vi "Begin.vi"(8 "error in":errorcluster) -> (0 "error out":errorcluster)   [LabVIEW 2017]
doc: "Called before other user functions, this VI is expected to open initial I/O refnums, load in file data, and do all program initialization. Notice that the <B>error out</B> terminal is simply used for data flow. Wiring it to other structures or subVIs ensures that this VI runs first."
uses:
  <vilib>/Rock Robotics/WPI/DriverStation/WPI_DriverStationRobotMode2.ctl
  <vilib>/Rock Robotics/WPI/Joystick/WPI_JoystickDeviceEnum.ctl
  <vilib>/Rock Robotics/WPI/Solenoid/WPI_SolenoidChannel.ctl
  <vilib>/Rock Robotics/SystemInterfaces/DIO/FPGA_DIORelayChannel.ctl
  <vilib>/Rock Robotics/WPI/Solenoid/WPI_SolenoidValue.ctl
  <vilib>/Rock Robotics/WPI/ThirdParty/Phoenix-LabVIEW/Motor Controller/Controls/CTRE_Phoenix_MotorControl_FeedbackDevice.ctl
  <vilib>/Rock Robotics/WPI/ThirdParty/Phoenix-LabVIEW/Motor Controller/Controls/CTRE_Phoenix_MotorControl_NeutralMode.ctl
  <vilib>/Rock Robotics/SystemInterfaces/AI/FPGA_AIChannel.ctl
  <vilib>/Rock Robotics/SystemInterfaces/DIO/FPGA_DIOChannel.ctl
  Robot Global Data.vi
  <vilib>/Rock Robotics/Network Tables/NT Write String Array.vi
  <vilib>/Rock Robotics/WPI/ThirdParty/Phoenix-LabVIEW/Pigeon IMU/CTRE_PigeonIMU_Open_TalonSRX.vi
  <vilib>/Rock Robotics/WPI/RobotDrive/WPI_RobotDriveOpen2MotorWithExistingMotors.vi
  <vilib>/Rock Robotics/WPI/Counter/WPI_CounterDigitalInputToDigitalSource.vi
  <vilib>/Rock Robotics/WPI/Solenoid/WPI_SolenoidOpenSingle.vi
  <vilib>/Rock Robotics/WPI/Solenoid/WPI_SolenoidOpenDouble.vi
  <vilib>/Rock Robotics/WPI/Utilities/WPI_GetSetVariantRefNum.vi
  <vilib>/Rock Robotics/WPI/Switch/WPI_SwitchOpenLimit.vi
  <vilib>/Rock Robotics/WPI/Solenoid/WPI_SolenoidSetEnum.vi
  <vilib>/Rock Robotics/WPI/ThirdParty/Phoenix-LabVIEW/Pigeon IMU/CTRE_PigeonIMU_Open_CAN.vi
  <vilib>/Rock Robotics/WPI/Ultrasonic/WPI_SonarMB1010DigRefNum Registry Set.vi
  <vilib>/Rock Robotics/SystemInterfaces/spilib/spi_bus.ctl
  <vilib>/Rock Robotics/WPI/Gyro/WPI_GyroXRS450_SPI_Open.vi
  <vilib>/Rock Robotics/WPI/Ultrasonic/WPI_SonarMB1010DigitalOpen.vi
panel:
  out "error out 3":errorcluster
  in  "error in 3":errorcluster
  out "error out 2":errorcluster
  in  "error in 2":errorcluster
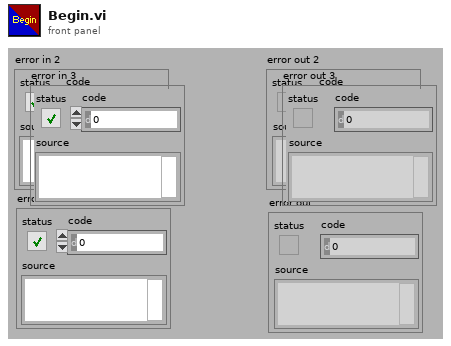
[diagram p1: front panel]
types:
  T1 = typedef "FPGA_DIOChannel.ctl" = enum8{"DIO 0", "DIO 1", "DIO 2", "DIO 3", "DIO 4", "DIO 5", "DIO 6", "DIO 7", "DIO 8", "DIO 9", "DIO MXP 0", "DIO MXP 1", "DIO MXP 2", "DIO MXP 3", "DIO MXP 4", "DIO MXP 5", "DIO MXP 6", "DIO MXP 7", "DIO MXP 8", "DIO MXP 9", "DIO MXP 10", "DIO MXP 11", "DIO MXP 12", "DIO MXP 13", "DIO MXP 14", "DIO MXP 15", "SPI Port CS1", "SPI Port CS2", "SPI Port CS3", "SPI Port MISO", "SPI Port MOSI", "Invalid"}
  T2 = typedef "WPI_JoystickDeviceEnum.ctl" = enum16{"USB 0", "USB 1", "USB 2", "USB 3", "USB 4", "USB 5"}
  T3 = typedef "WPI_SolenoidChannel.ctl" = enum8{"Solenoid 0", "Solenoid 1", "Solenoid 2", "Solenoid 3", "Solenoid 4", "Solenoid 5", "Solenoid 6", "Solenoid 7", "Invalid"}
  T4 = typedef "WPI_DriverStationRobotMode2.ctl" = enum16{"Autonomous Disabled", "Autonomous Enabled", "Teleop Disabled", "Teleop Enabled", "Disconnected", "Finish", "Test Disabled", "Test Enabled", "Emergency Stopped"}
  T5 = typedef "FPGA_AIChannel.ctl" = enum8{"AI 0", "AI 1", "AI 2", "AI 3", "AI MXP 0", "AI MXP 1", "AI MXP 2", "AI MXP 3", "Invalid"}
  T6 = typedef "CTRE_Phoenix_MotorControl_NeutralMode.ctl" = enum8{"EEPROMSetting", "Override to Coast", "Override to Brake"}
  T7 = typedef "WPI_SolenoidValue.ctl" = enum16{"Off", "On", "Forward", "Reverse"}
  T8 = typedef "FPGA_DIORelayChannel.ctl" = enum8{"Relay 0", "Relay 1", "Relay 2", "Relay 3", "Invalid"}
  T9 = typedef "spi_bus.ctl" = enum16{"SPI On-Board, CS0", "SPI On-Board, CS1", "SPI On-Board, CS2", "SPI On-Board, CS3", "SPI MXP", "Invalid"}
  T10 = typedef "WPI_JoystickDevRef.ctl" = cluster{"Device":T2}
  T11 = typedef "WPI_DigitalInputDevRef.ctl" = cluster{"DevStatus":errorcluster, "DIO Channel":T1}
  T12 = typedef "FPGA_CounterEncoderSourceConvertionLVSourceType.ctl" = cluster{"DevStatus":errorcluster, "AnalogTriggerMode?":bool, "DigitalMode":cluster{"DIO Channel":T13}, "AnalogTriggerMode":cluster{"AnalogTriggerIndex":T14, "OutputType":T15}}
  T13 = typedef "FPGA_DIODigitalSourceChannel.ctl" = enum8{"DIO 0", "DIO 1", "DIO 2", "DIO 3", "DIO 4", "DIO 5", "DIO 6", "DIO 7", "DIO 8", "DIO 9", "DIO MXP 0", "DIO MXP 1", "DIO MXP 2", "DIO MXP 3", "DIO MXP 4", "DIO MXP 5", "DIO MXP 6", "DIO MXP 7", "DIO MXP 8", "DIO MXP 9", "DIO MXP 10", "DIO MXP 11", "DIO MXP 12", "DIO MXP 13", "DIO MXP 14", "DIO MXP 15", "Disabled"}
  T14 = typedef "FPGA_AnalogTriggerIndex.ctl" = enum8{"Trig 0", "Trig 1", "Trig 2", "Trig 3", "Trig 4", "Trig 5", "Trig 6", "Trig 7", "Invalid"}
  T15 = typedef "FPGA_AnalogTriggerOutType.ctl" = enum16{"InWindow", "TriggerState", "Rising", "Falling"}
  T16 = typedef "WPI_EncoderDevRef.ctl" = cluster{"DevStatus":errorcluster, "EncoderIndex":T17, "CounterIndex":T18, "DistancePerCount":dbl, "Decoding Type":T19}
  T17 = typedef "FPGA_EncoderIdx.ctl" = enum8{"Enc 0", "Enc 1", "Enc 2", "Enc 3", "Enc 4", "Enc 5", "Enc 6", "Enc 7", "Invalid"}
  T18 = typedef "FPGA_CounterCtrSystemIndex.ctl" = enum8{"Ctr 0", "Ctr 1", "Ctr 2", "Ctr 3", "Ctr 4", "Ctr 5", "Ctr 6", "Ctr 7", "Invalid"}
  T19 = typedef "WPI_EncoderType.ctl" = enum16{"1x", "2x", "4x"}
  T20 = typedef "WPI_SolenoidDevRef.ctl" = cluster{"DevStatus":errorcluster, "Pneumatics Control Module":u8, "Forward Solenoid Channel":T3, "Reverse Solenoid Channel":T3}
  T21 = typedef "WPI_CompressorDevRef.ctl" = cluster{"DevStatus":errorcluster, "Pneumatics Control Module":u8}
  T22 = typedef "WPI_SwitchDevRef.ctl" = cluster{"DevStatus":errorcluster, "DIO Channel":T1, "CntIndex":T18, "Normally Closed":bool}
  T23 = typedef "WPI_MotorControlDeviceRef.ctl" = cluster{"DeviceStatus":errorcluster, "Type":T24, "PWM":cluster{"PWM Channel":T25, "DeadBand":T26}, "CAN":cluster{"Device Number":u8, "SetOutput VI Ref":variant, "GetOutput VI Ref":variant, "Enable VI Ref":variant, "Disable VI Ref":variant, "Data":variant}, "Invert":bool, "DIO PWM":cluster{"PWM \"Enable\" Channel":T25, "DIOChannel":T1, "PWM Rate":dbl}}
  T24 = typedef "WPI_MotorControlType.ctl" = enum16{"PWM", "CAN", "DIO PWM"}
  T25 = typedef "FPGA_DIOPWMChannel.ctl" = enum8{"PWM 0", "PWM 1", "PWM 2", "PWM 3", "PWM 4", "PWM 5", "PWM 6", "PWM 7", "PWM 8", "PWM 9", "PWM MXP 0", "PWM MXP 1", "PWM MXP 2", "PWM MXP 3", "PWM MXP 4", "PWM MXP 5", "PWM MXP 6", "PWM MXP 7", "PWM MXP 8", "PWM MXP 9", "Invalid"}
  T26 = typedef "WPI_PWMDeadband.ctl" = cluster{"Name":string, "maxPositivePwm":i32, "minPositivePwm":i32, "centerPwm":i32, "maxNegativePwm":i32, "minNegativePwm":i32, "angularRange":u16}
  T27 = typedef "WPI_RobotDriveDevRef.ctl" = cluster{"DevStatus":errorcluster, "Motors[]":T23[], "Square Inputs":bool, "Max Output":dbl}
  T28 = typedef "CTRE_PigeonIMU_DeviceRef.ctl" = cluster{"DeviceStatus":errorcluster, "Device Number":u8, "Type":T29, "Device ID":u32, "Handle":u64, "UsageFrame":u32, "Library Path":path}
  T29 = typedef "CTRE_PigeonIMU_ConnectionType.ctl" = u32
  T30 = typedef "CTRE_Phoenix_MotorControl_FeedbackDevice.ctl" = i8
  T31 = typedef "WPI_AnalogChannelDevRef.ctl" = cluster{"DevStatus":errorcluster, "Analog Channel":T5}
  T32 = typedef "WPI_SonarMB1010DigitalDeviceRef.ctl" = cluster{"CounterDevRef":T33, "Scaling factor (s/in)":dbl}
  T33 = typedef "WPI_CounterDevRef.ctl" = cluster{"DevStatus":errorcluster, "CntIndex":T18}
  T34 = typedef "WPI_RelayDevRef.ctl" = cluster{"DevStatus":errorcluster, "Relay Channel":T8, "Relay Direction":T35}
  T35 = typedef "WPI_RelayDirection.ctl" = enum16{"Both directions", "Forward only", "Reverse only"}
  T36 = typedef "WPI_GyroDevRef.ctl" = cluster{"DevStatus":errorcluster, "Analog Channel":T5, "Gain (VoltsPerDegree/Second)":dbl, "Gyro Type":enum16{"Analog", "XRS450"}, "Handle":i32, "SPI Bus":T9, "Device Found":bool, "Sample Rate":dbl, "Calibrate On Open":bool, "Offset":dbl}
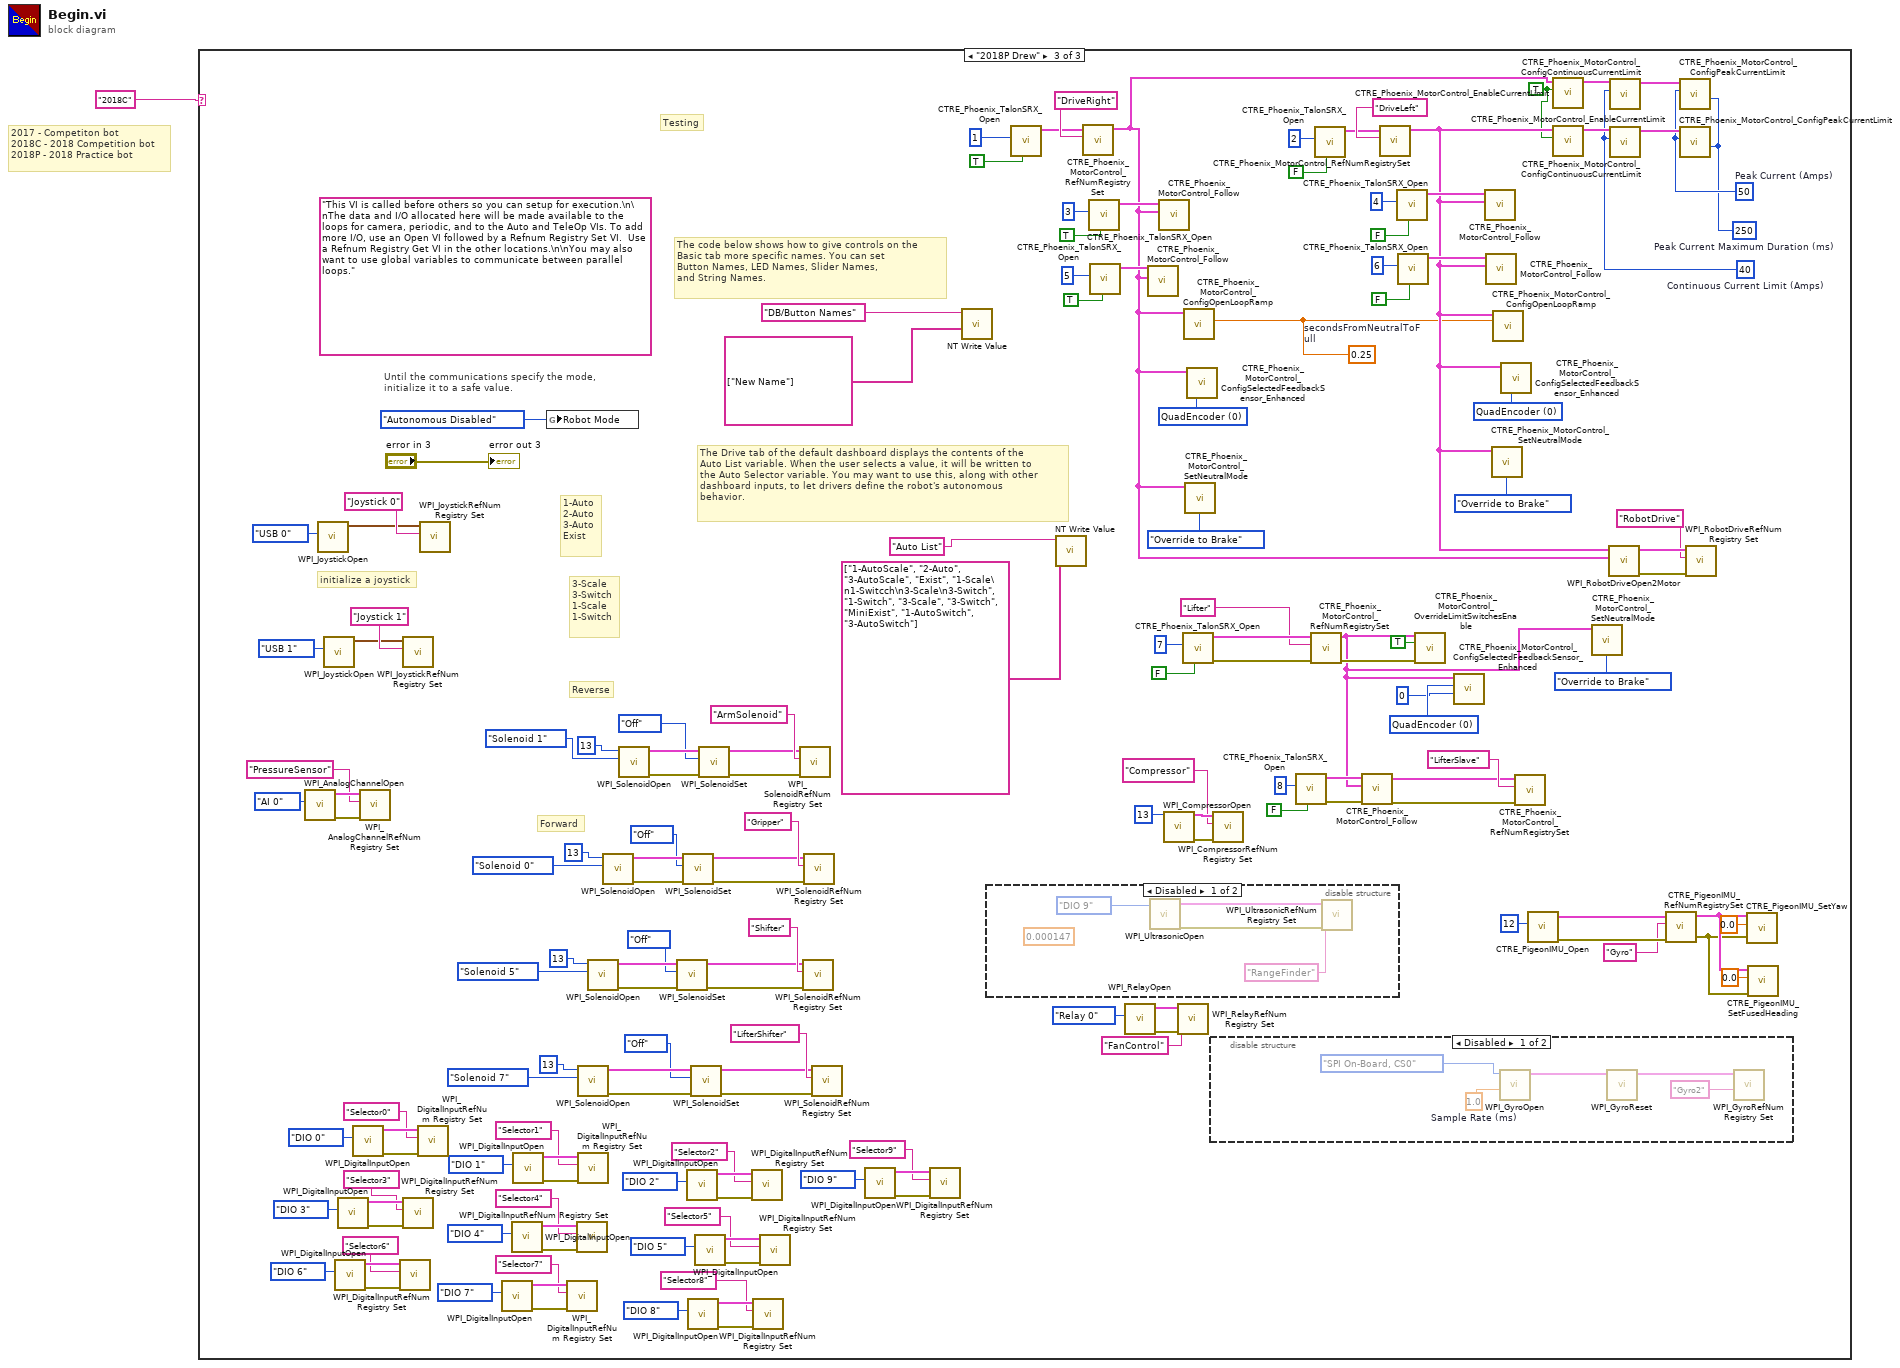
[diagram p0: block diagram]
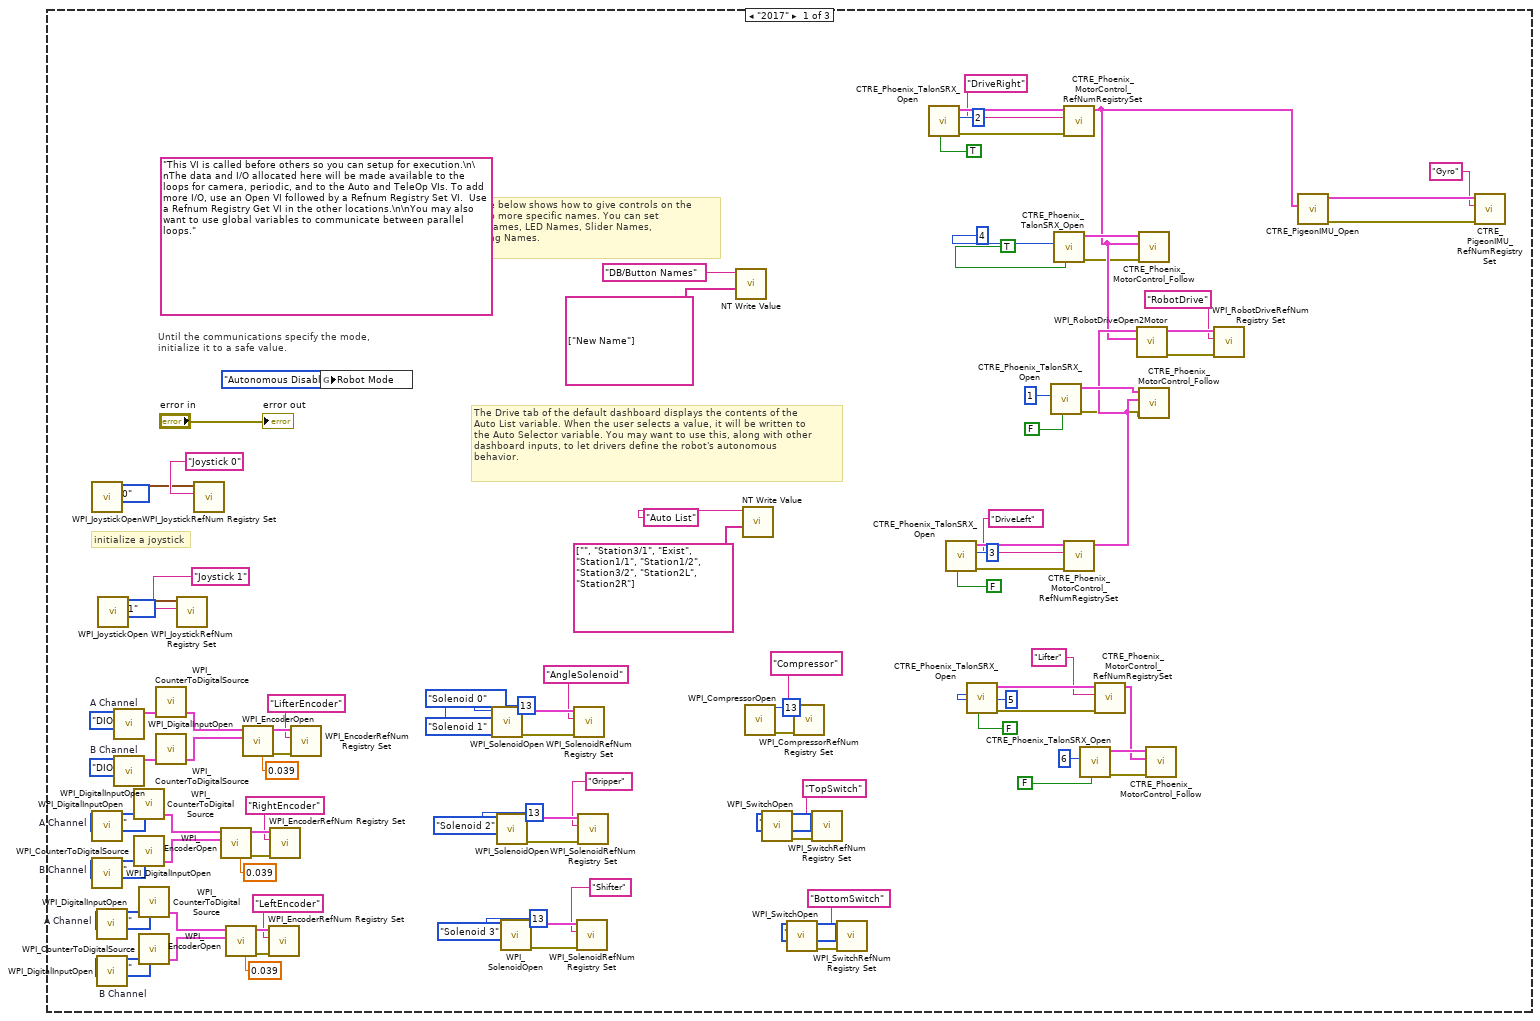
[diagram p2: hidden frame]
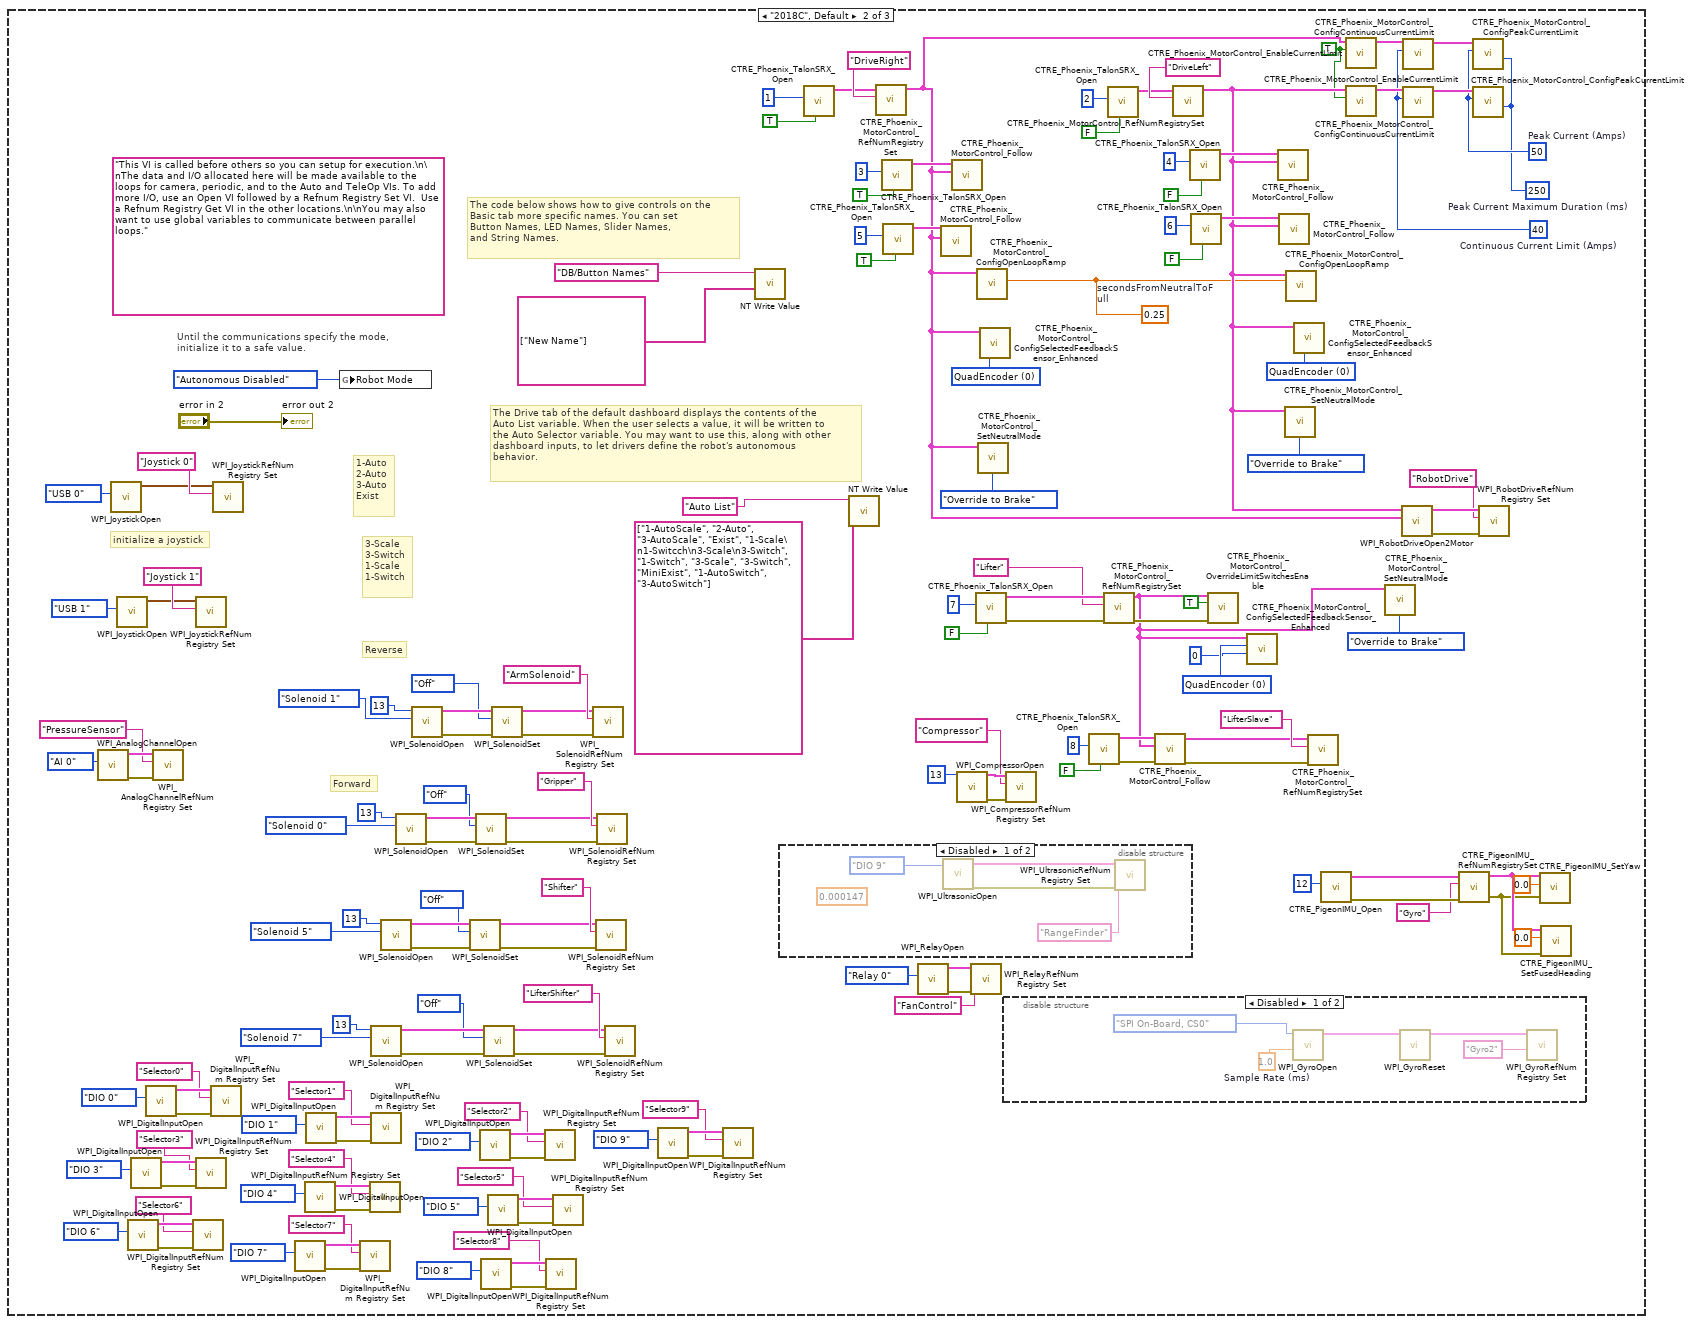
[diagram p3: hidden frame]
diagram:
  # "2017 - Competiton bot\n2018C - 2018 Competition bot\n2018P - 2018 Practice bot"
  n1 = case shown="\"2018P Drew\"" "2018C" {
    frame "2017" {
      w34 = FPGA_DIOChannel."DIO 5"  # B Channel
      w33 = FPGA_DIOChannel."DIO 4"  # A Channel
      w69 = FPGA_DIOChannel."DIO 3"  # B Channel
      w68 = FPGA_DIOChannel."DIO 2"  # A Channel
      w79 = FPGA_DIOChannel."DIO 1"  # B Channel
      w78 = FPGA_DIOChannel."DIO 0"  # A Channel
      (unwired) "This VI is called before others so you can setup for execution.\n\nThe data and I/O allocated here will be made available to the loops for camera, periodic, and to the Auto and TeleOp VIs. To add more I/O, use an Open VI followed by a Refnum Registry Set VI.  Use a Refnum Registry Get VI in the other locations.\n\nYou may also want to use global variables to communicate between parallel loops."
      # "The Drive tab of the default dashboard displays the contents of the\nAuto List variable. When the user selects a value, it will be written to\nthe Auto Selector variable. You may want to use this, along with other\ndashboard inputs, to let drivers define the robot's autonomous\nbehavior."
      # "The code below shows how to give controls on the\nBasic tab more specific names. You can set\nButton Names, LED Names, Slider Names,\nand String Names."
      # "initialize a joystick"
      # "Until the communications specify the mode,\ninitialize it to a safe value."
      n2 = call <vilib>:"WPI_JoystickOpen.vi"("JoystickDevice"=WPI_JoystickDeviceEnum."USB 0") -> ("JoystickDevRef"=w105:T10)  [unwired: 10 in]
      n3 = call <vilib>:"WPI_DigitalInputOpen.vi"("DIO Channel"=w78) -> ("DigitalInputDevRef"=w75:T11)  [unwired: 1 in, 9 out]
      n4 = call <vilib>:"WPI_DigitalInputOpen.vi"("DIO Channel"=w79) -> ("DigitalInputDevRef"=w76:T11)  [unwired: 1 in, 9 out]
      n5 = call <vilib>:"WPI_DigitalInputOpen.vi"("DIO Channel"=w68) -> ("DigitalInputDevRef"=w65:T11)  [unwired: 1 in, 9 out]
      n6 = call <vilib>:"WPI_DigitalInputOpen.vi"("DIO Channel"=w69) -> ("DigitalInputDevRef"=w66:T11)  [unwired: 1 in, 9 out]
      n7 = call <vilib>:"WPI_JoystickOpen.vi"("JoystickDevice"=WPI_JoystickDeviceEnum."USB 1") -> ("JoystickDevRef"=w36:T10)  [unwired: 10 in]
      n8 = call <vilib>:"WPI_DigitalInputOpen.vi"("DIO Channel"=w33) -> ("DigitalInputDevRef"=w30:T11)  [unwired: 1 in, 9 out]
      n9 = call <vilib>:"WPI_DigitalInputOpen.vi"("DIO Channel"=w34) -> ("DigitalInputDevRef"=w31:T11)  [unwired: 1 in, 9 out]
      n10 = call-poly <vilib>:"WPI_CounterToDigitalSource.vi"("DigitalInputDevRef"=w75) -> ("Digital Source"=w74:T12)  [unwired: 6 out]
      n11 = call-poly <vilib>:"WPI_CounterToDigitalSource.vi"("DigitalInputDevRef"=w76) -> ("Digital Source"=w77:T12)  [unwired: 6 out]
      n12 = call-poly <vilib>:"WPI_CounterToDigitalSource.vi"("DigitalInputDevRef"=w65) -> ("Digital Source"=w64:T12)  [unwired: 6 out]
      n13 = call-poly <vilib>:"WPI_CounterToDigitalSource.vi"("DigitalInputDevRef"=w66) -> ("Digital Source"=w67:T12)  [unwired: 6 out]
      n14 = call-poly <vilib>:"WPI_CounterToDigitalSource.vi"("DigitalInputDevRef"=w30) -> ("Digital Source"=w29:T12)  [unwired: 6 out]
      n15 = call-poly <vilib>:"WPI_CounterToDigitalSource.vi"("DigitalInputDevRef"=w31) -> ("Digital Source"=w32:T12)  [unwired: 6 out]
      n16 = call <vilib>:"WPI_JoystickRefNum Registry Set.vi"("refnum name"="Joystick 1", "JoystickDevRef"=w36) -> ()  [unwired: 8 in, 2 out]
      n17 = call <vilib>:"WPI_JoystickRefNum Registry Set.vi"("refnum name"="Joystick 0", "JoystickDevRef"=w105) -> ()  [unwired: 8 in, 2 out]
      n18 = call <vilib>:"WPI_EncoderOpen.vi"("DistancePerCount"=0.039, "BSource"=w77, "ASource"=w74) -> ("error out"=w73:errorcluster, "EncoderDevRef"=w72:T16)  [unwired: 5 in, 2 out]
      n19 = call <vilib>:"WPI_EncoderOpen.vi"("DistancePerCount"=0.039, "BSource"=w67, "ASource"=w64) -> ("error out"=w63:errorcluster, "EncoderDevRef"=w62:T16)  [unwired: 5 in, 2 out]
      n20 = call <vilib>:"WPI_EncoderOpen.vi"("DistancePerCount"=0.039, "BSource"=w32, "ASource"=w29) -> ("error out"=w28:errorcluster, "EncoderDevRef"=w27:T16)  [unwired: 5 in, 2 out]
      n21 = call <vilib>:"WPI_EncoderRefNum Registry Set.vi"("error in (no error)"=w63, "refnum name"="LeftEncoder", "EncoderDevRef"=w62) -> ()  [unwired: 7 in, 2 out]
      n22 = call <vilib>:"WPI_EncoderRefNum Registry Set.vi"("error in (no error)"=w73, "refnum name"="RightEncoder", "EncoderDevRef"=w72) -> ()  [unwired: 7 in, 2 out]
      n23 = call <vilib>:"WPI_EncoderRefNum Registry Set.vi"("error in (no error)"=w28, "refnum name"="LifterEncoder", "EncoderDevRef"=w27) -> ()  [unwired: 7 in, 2 out]
      n24 = global write "Robot Global Data.vi" "Robot Mode"(WPI_DriverStationRobotMode2."Autonomous Disabled" ("Robot Mode")) -> ()
      n25 = call-poly <vilib>:"WPI_SolenoidOpen.vi"("Reverse Solenoid Channel"=WPI_SolenoidChannel."Solenoid 1", "Forward Solenoid Channel"=WPI_SolenoidChannel."Solenoid 0", "Pneumatics Control Module (0)"=u8 13) -> ("error out"=w59:errorcluster, "SolenoidDevRef"=w58:T20)  [unwired: 7 in]
      n26 = call-poly <vilib>:"WPI_SolenoidOpen.vi"("Solenoid Channel"=WPI_SolenoidChannel."Solenoid 2" ("Forward Solenoid Channel"), "Pneumatics Control Module (0)"=u8 13) -> ("error out"=w54:errorcluster, "SolenoidDevRef"=w53:T20)  [unwired: 8 in]
      n27 = call-poly <vilib>:"WPI_SolenoidOpen.vi"("Solenoid Channel"=WPI_SolenoidChannel."Solenoid 3" ("Forward Solenoid Channel"), "Pneumatics Control Module (0)"=u8 13) -> ("error out"=w50:errorcluster, "SolenoidDevRef"=w49:T20)  [unwired: 8 in]
      n28 = call <vilib>:"WPI_SolenoidRefNum Registry Set.vi"("error in (no error)"=w59, "refnum name"="AngleSolenoid", "SolenoidDevRef"=w58) -> ()  [unwired: 7 in, 2 out]
      n29 = call <vilib>:"WPI_SolenoidRefNum Registry Set.vi"("error in (no error)"=w50, "refnum name"="Shifter", "SolenoidDevRef"=w49) -> ()  [unwired: 7 in, 2 out]
      n30 = call <vilib>:"WPI_SolenoidRefNum Registry Set.vi"("error in (no error)"=w54, "refnum name"="Gripper", "SolenoidDevRef"=w53) -> ()  [unwired: 7 in, 2 out]
      n31 = call-poly <vilib>:"NT Write Value.vi"("String Array"=string[] ["New Name"], "Name"="DB/Button Names") -> ()  [unwired: 9 in, 1 out]
      n32 = call-poly <vilib>:"NT Write Value.vi"("String Array"=string[] ["", "Station3/1", "Exist", "Station1/1", "Station1/2", "Station3/2", "Station2L", "Station2R"], "Name"="Auto List") -> ()  [unwired: 9 in, 1 out]
      n33 = call <vilib>:"WPI_CompressorOpen.vi"("Pneumatics Control Module (0)"=u8 13) -> ("CompressorDevRef"=w41:T21, "error out"=w42:errorcluster)  [unwired: 13 in]
      n34 = call-poly <vilib>:"WPI_SwitchOpen.vi"("DIO Channel"=FPGA_DIOChannel."DIO 0") -> ("error out"=w15:errorcluster, "SwitchDevRef"=w14:T22)  [unwired: 9 in]
      n35 = call-poly <vilib>:"WPI_SwitchOpen.vi"("DIO Channel"=FPGA_DIOChannel."DIO 0") -> ("error out"=w11:errorcluster, "SwitchDevRef"=w10:T22)  [unwired: 9 in]
      n36 = call <vilib>:"WPI_CompressorRefNum Registry Set.vi"("error in (no error)"=w42, "refnum name"="Compressor", "CompressorDevRef"=w41) -> ()  [unwired: 7 in, 2 out]
      n37 = call <vilib>:"WPI_SwitchRefNum Registry Set.vi"("error in (no error)"=w15, "refnum name"="TopSwitch", "SwitchDevRef"=w14) -> ()  [unwired: 7 in, 2 out]
      n38 = call <vilib>:"WPI_SwitchRefNum Registry Set.vi"("error in (no error)"=w11, "refnum name"="BottomSwitch", "SwitchDevRef"=w10) -> ()  [unwired: 7 in, 2 out]
      n39 = call <vilib>:"CTRE_Phoenix_TalonSRX_Open.vi"("Invert"=TRUE, "Device Number"=u8 2) -> ("error out"=w93:errorcluster, "CAN Talon SRX Ref"=w92:T23)  [unwired: 8 in]
      n40 = call <vilib>:"CTRE_Phoenix_TalonSRX_Open.vi"("Invert"=FALSE, "Device Number"=u8 3) -> ("error out"=w98:errorcluster, "CAN Talon SRX Ref"=w97:T23)  [unwired: 8 in]
      n41 = call <vilib>:"CTRE_Phoenix_TalonSRX_Open.vi"("Invert"=FALSE, "Device Number"=u8 5) -> ("error out"=w24:errorcluster, "CAN Talon SRX Ref"=w23:T23)  [unwired: 8 in]
      n42 = call <vilib>:"CTRE_Phoenix_TalonSRX_Open.vi"("Invert"=FALSE, "Device Number"=u8 1) -> ("error out"=w6:errorcluster, "CAN Talon SRX Ref"=w81:T23)  [unwired: 8 in]
      n43 = call <vilib>:"CTRE_Phoenix_TalonSRX_Open.vi"("Invert"=TRUE, "Device Number"=u8 4) -> ("error out"=w5:errorcluster, "CAN Talon SRX Ref"=w39:T23)  [unwired: 8 in]
      n44 = call <vilib>:"CTRE_Phoenix_MotorControl_RefNumRegistrySet.vi"("error in (no error)"=w93, "refnum name"="DriveRight", "PhoenixMotorControlDevRef"=w92) -> ("PhoenixMotorControlDevRef"=w38:T23)  [unwired: 7 in, 1 out]
      n45 = call <vilib>:"CTRE_Phoenix_MotorControl_RefNumRegistrySet.vi"("error in (no error)"=w98, "refnum name"="DriveLeft", "PhoenixMotorControlDevRef"=w97) -> ("PhoenixMotorControlDevRef"=w80:T23)  [unwired: 7 in, 1 out]
      n46 = call <vilib>:"CTRE_Phoenix_TalonSRX_Open.vi"("Invert"=FALSE, "Device Number"=u8 6) -> ("error out"=w19:errorcluster, "CAN Talon SRX Ref"=w18:T23)  [unwired: 8 in]
      n47 = call <vilib>:"CTRE_Phoenix_MotorControl_RefNumRegistrySet.vi"("error in (no error)"=w24, "refnum name"="Lifter", "PhoenixMotorControlDevRef"=w23) -> ("PhoenixMotorControlDevRef"=w7:T23)  [unwired: 7 in, 1 out]
      n48 = call-poly <vilib>:"WPI_RobotDriveOpen2Motor.vi"("Right Motor Dev Ref"=w38, "Left Motor Dev Ref"=w80) -> ("error out"=w88:errorcluster, "RobotDriveDevRef"=w87:T27)  [unwired: 8 in]
      n49 = call <vilib>:"CTRE_Phoenix_MotorControl_Follow.vi"("error in (no error)"=w5, "Master Controller to Follow"=w38, "PhoenixMotorControlDevRef"=w39) -> ()  [unwired: 7 in, 2 out]
      n50 = call <vilib>:"CTRE_Phoenix_MotorControl_Follow.vi"("error in (no error)"=w6, "Master Controller to Follow"=w80, "PhoenixMotorControlDevRef"=w81) -> ()  [unwired: 7 in, 2 out]
      n51 = call <vilib>:"CTRE_Phoenix_MotorControl_Follow.vi"("error in (no error)"=w19, "Master Controller to Follow"=w7, "PhoenixMotorControlDevRef"=w18) -> ()  [unwired: 7 in, 2 out]
      n52 = call <vilib>:"WPI_RobotDriveRefNum Registry Set.vi"("error in (no error)"=w88, "refnum name"="RobotDrive", "RobotDriveDevRef"=w87) -> ()  [unwired: 7 in, 2 out]
      n53 = call-poly <vilib>:"CTRE_PigeonIMU_Open.vi"("CAN Talon SRX Ref"=w38) -> ("error out"=w4:errorcluster, "PigeonIMUDevRef"=w3:T28)  [unwired: 9 in]
      n54 = call <vilib>:"CTRE_PigeonIMU_RefNumRegistrySet.vi"("error in (no error)"=w4, "refnum name"="Gyro", "PigeonIMUDevRef"=w3) -> ()  [unwired: 7 in, 2 out]
      "error out" <- "error in"
    }
    frame "2018C", Default {
      w158 = 250  # Peak Current Maximum Duration (ms)
      w159 = 50  # Peak Current (Amps)
      w160 = 40  # Continuous Current Limit (Amps)
      w155 = TRUE ("Enable Current Limit?")
      w174 = T30 0 items=["None"=-1, "QuadEncoder"=0, "Analog"=2, "Tachometer"=4, "Pulse Width Encoded Position"=8, "Sensor Sum (S0 + S1)"=9, "Sensor Difference (D0 - D1)"=10, "Remote Source 0"=11, "Remote Source 1"=12, "Software Emulated"=15] ("Feedback Device")
      w175 = T30 0 items=["None"=-1, "QuadEncoder"=0, "Analog"=2, "Tachometer"=4, "Pulse Width Encoded Position"=8, "Sensor Sum (S0 + S1)"=9, "Sensor Difference (D0 - D1)"=10, "Remote Source 0"=11, "Remote Source 1"=12, "Software Emulated"=15] ("Feedback Device")
      w176 = T30 0 items=["None"=-1, "QuadEncoder"=0, "Analog"=2, "Tachometer"=4, "Pulse Width Encoded Position"=8, "Sensor Sum (S0 + S1)"=9, "Sensor Difference (D0 - D1)"=10, "Remote Source 0"=11, "Remote Source 1"=12, "Software Emulated"=15] ("Feedback Device")
      w154 = 0.25  # secondsFromNeutralToFull
      (unwired) "This VI is called before others so you can setup for execution.\n\nThe data and I/O allocated here will be made available to the loops for camera, periodic, and to the Auto and TeleOp VIs. To add more I/O, use an Open VI followed by a Refnum Registry Set VI.  Use a Refnum Registry Get VI in the other locations.\n\nYou may also want to use global variables to communicate between parallel loops."
      # "1-Auto\n2-Auto\n3-Auto\nExist"
      # "3-Scale\n3-Switch\n1-Scale\n1-Switch"
      # "Forward"
      # "Reverse"
      # "The Drive tab of the default dashboard displays the contents of the\nAuto List variable. When the user selects a value, it will be written to\nthe Auto Selector variable. You may want to use this, along with other\ndashboard inputs, to let drivers define the robot's autonomous\nbehavior."
      # "The code below shows how to give controls on the\nBasic tab more specific names. You can set\nButton Names, LED Names, Slider Names,\nand String Names."
      # "initialize a joystick"
      # "Until the communications specify the mode,\ninitialize it to a safe value."
      n55 = call <vilib>:"WPI_AnalogChannelOpen.vi"("Analog Channel"=FPGA_AIChannel."AI 0") -> ("error out"=w150:errorcluster, "AIDeviceRef"=w151:T31)  [unwired: 9 in]
      n56 = call <vilib>:"WPI_JoystickOpen.vi"("JoystickDevice"=WPI_JoystickDeviceEnum."USB 0") -> ("JoystickDevRef"=w261:T10)  [unwired: 10 in]
      n57 = call <vilib>:"WPI_JoystickOpen.vi"("JoystickDevice"=WPI_JoystickDeviceEnum."USB 1") -> ("JoystickDevRef"=w217:T10)  [unwired: 10 in]
      n58 = call <vilib>:"WPI_DigitalInputOpen.vi"("DIO Channel"=FPGA_DIOChannel."DIO 6") -> ("error out"=w140:errorcluster, "DigitalInputDevRef"=w139:T11)  [unwired: 9 in]
      n59 = call <vilib>:"WPI_DigitalInputOpen.vi"("DIO Channel"=FPGA_DIOChannel."DIO 3") -> ("error out"=w143:errorcluster, "DigitalInputDevRef"=w142:T11)  [unwired: 9 in]
      n60 = call <vilib>:"WPI_DigitalInputOpen.vi"("DIO Channel"=FPGA_DIOChannel."DIO 0") -> ("error out"=w146:errorcluster, "DigitalInputDevRef"=w145:T11)  [unwired: 9 in]
      n61 = call <vilib>:"WPI_AnalogChannelRefNum Registry Set.vi"("error in (no error)"=w150, "refnum name"="PressureSensor", "AIDeviceRef"=w151) -> ()  [unwired: 7 in, 2 out]
      n62 = call <vilib>:"WPI_DigitalInputRefNum Registry Set.vi"("error in (no error)"=w140, "refnum name"="Selector6", "DigitalInputDevRef"=w139) -> ()  [unwired: 7 in, 2 out]
      n63 = call <vilib>:"WPI_JoystickRefNum Registry Set.vi"("refnum name"="Joystick 1", "JoystickDevRef"=w217) -> ()  [unwired: 8 in, 2 out]
      n64 = call <vilib>:"WPI_DigitalInputRefNum Registry Set.vi"("error in (no error)"=w143, "refnum name"="Selector3", "DigitalInputDevRef"=w142) -> ()  [unwired: 7 in, 2 out]
      n65 = call <vilib>:"WPI_DigitalInputRefNum Registry Set.vi"("error in (no error)"=w146, "refnum name"="Selector0", "DigitalInputDevRef"=w145) -> ()  [unwired: 7 in, 2 out]
      n66 = call <vilib>:"WPI_JoystickRefNum Registry Set.vi"("refnum name"="Joystick 0", "JoystickDevRef"=w261) -> ()  [unwired: 8 in, 2 out]
      n67 = call <vilib>:"WPI_DigitalInputOpen.vi"("DIO Channel"=FPGA_DIOChannel."DIO 7") -> ("error out"=w137:errorcluster, "DigitalInputDevRef"=w136:T11)  [unwired: 9 in]
      n68 = call <vilib>:"WPI_DigitalInputOpen.vi"("DIO Channel"=FPGA_DIOChannel."DIO 4") -> ("error out"=w134:errorcluster, "DigitalInputDevRef"=w133:T11)  [unwired: 9 in]
      n69 = call <vilib>:"WPI_DigitalInputOpen.vi"("DIO Channel"=FPGA_DIOChannel."DIO 1") -> ("error out"=w131:errorcluster, "DigitalInputDevRef"=w130:T11)  [unwired: 9 in]
      n70 = global write "Robot Global Data.vi" "Robot Mode"(WPI_DriverStationRobotMode2."Autonomous Disabled" ("Robot Mode")) -> ()
      n71 = call <vilib>:"WPI_DigitalInputRefNum Registry Set.vi"("error in (no error)"=w137, "refnum name"="Selector7", "DigitalInputDevRef"=w136) -> ()  [unwired: 7 in, 2 out]
      n72 = call <vilib>:"WPI_DigitalInputRefNum Registry Set.vi"("error in (no error)"=w134, "refnum name"="Selector4", "DigitalInputDevRef"=w133) -> ()  [unwired: 7 in, 2 out]
      n73 = call-poly <vilib>:"WPI_SolenoidOpen.vi"("Solenoid Channel"=WPI_SolenoidChannel."Solenoid 7" ("Forward Solenoid Channel"), "Pneumatics Control Module (0)"=u8 13) -> ("error out"=w206:errorcluster, "SolenoidDevRef"=w205:T20)  [unwired: 8 in]
      n74 = call <vilib>:"WPI_DigitalInputRefNum Registry Set.vi"("error in (no error)"=w131, "refnum name"="Selector1", "DigitalInputDevRef"=w130) -> ()  [unwired: 7 in, 2 out]
      n75 = call-poly <vilib>:"WPI_SolenoidOpen.vi"("Solenoid Channel"=WPI_SolenoidChannel."Solenoid 5" ("Forward Solenoid Channel"), "Pneumatics Control Module (0)"=u8 13) -> ("error out"=w233:errorcluster, "SolenoidDevRef"=w232:T20)  [unwired: 8 in]
      n76 = call-poly <vilib>:"WPI_SolenoidOpen.vi"("Solenoid Channel"=WPI_SolenoidChannel."Solenoid 0" ("Forward Solenoid Channel"), "Pneumatics Control Module (0)"=u8 13) -> ("error out"=w237:errorcluster, "SolenoidDevRef"=w236:T20)  [unwired: 8 in]
      n77 = call-poly <vilib>:"WPI_SolenoidOpen.vi"("Solenoid Channel"=WPI_SolenoidChannel."Solenoid 1" ("Forward Solenoid Channel"), "Pneumatics Control Module (0)"=u8 13) -> ("error out"=w241:errorcluster, "SolenoidDevRef"=w240:T20)  [unwired: 8 in]
      n78 = call-poly <vilib>:"WPI_SolenoidSet.vi"("Value"=WPI_SolenoidValue."Off", "SolenoidDevRef"=w232) -> ("SolenoidDevRef"=w182:T20)  [unwired: 8 in, 1 out]
      n79 = call-poly <vilib>:"WPI_SolenoidSet.vi"("Value"=WPI_SolenoidValue."Off", "SolenoidDevRef"=w236) -> ("SolenoidDevRef"=w186:T20)  [unwired: 8 in, 1 out]
      n80 = call <vilib>:"WPI_DigitalInputOpen.vi"("DIO Channel"=FPGA_DIOChannel."DIO 2") -> ("error out"=w128:errorcluster, "DigitalInputDevRef"=w127:T11)  [unwired: 9 in]
      n81 = call <vilib>:"WPI_DigitalInputOpen.vi"("DIO Channel"=FPGA_DIOChannel."DIO 8") -> ("error out"=w122:errorcluster, "DigitalInputDevRef"=w121:T11)  [unwired: 9 in]
      n82 = call-poly <vilib>:"WPI_SolenoidSet.vi"("Value"=WPI_SolenoidValue."Off", "SolenoidDevRef"=w205) -> ("SolenoidDevRef"=w181:T20)  [unwired: 8 in, 1 out]
      n83 = call <vilib>:"WPI_DigitalInputOpen.vi"("DIO Channel"=FPGA_DIOChannel."DIO 5") -> ("error out"=w125:errorcluster, "DigitalInputDevRef"=w124:T11)  [unwired: 9 in]
      n84 = call-poly <vilib>:"WPI_SolenoidSet.vi"("Value"=WPI_SolenoidValue."Off", "SolenoidDevRef"=w240) -> ("SolenoidDevRef"=w185:T20)  [unwired: 8 in, 1 out]
      n85 = call <vilib>:"WPI_DigitalInputRefNum Registry Set.vi"("error in (no error)"=w128, "refnum name"="Selector2", "DigitalInputDevRef"=w127) -> ()  [unwired: 7 in, 2 out]
      n86 = call <vilib>:"WPI_DigitalInputRefNum Registry Set.vi"("error in (no error)"=w122, "refnum name"="Selector8", "DigitalInputDevRef"=w121) -> ()  [unwired: 7 in, 2 out]
      n87 = call <vilib>:"WPI_DigitalInputRefNum Registry Set.vi"("error in (no error)"=w125, "refnum name"="Selector5", "DigitalInputDevRef"=w124) -> ()  [unwired: 7 in, 2 out]
      n88 = call <vilib>:"WPI_SolenoidRefNum Registry Set.vi"("error in (no error)"=w241, "refnum name"="ArmSolenoid", "SolenoidDevRef"=w185) -> ()  [unwired: 7 in, 2 out]
      n89 = call <vilib>:"WPI_SolenoidRefNum Registry Set.vi"("error in (no error)"=w233, "refnum name"="Shifter", "SolenoidDevRef"=w182) -> ()  [unwired: 7 in, 2 out]
      n90 = call <vilib>:"WPI_SolenoidRefNum Registry Set.vi"("error in (no error)"=w237, "refnum name"="Gripper", "SolenoidDevRef"=w186) -> ()  [unwired: 7 in, 2 out]
      n91 = call <vilib>:"WPI_SolenoidRefNum Registry Set.vi"("error in (no error)"=w206, "refnum name"="LifterShifter", "SolenoidDevRef"=w181) -> ()  [unwired: 7 in, 2 out]
      n92 = call <vilib>:"WPI_DigitalInputOpen.vi"("DIO Channel"=FPGA_DIOChannel."DIO 9") -> ("error out"=w110:errorcluster, "DigitalInputDevRef"=w109:T11)  [unwired: 9 in]
      n93 = call <vilib>:"WPI_DigitalInputRefNum Registry Set.vi"("error in (no error)"=w110, "refnum name"="Selector9", "DigitalInputDevRef"=w109) -> ()  [unwired: 7 in, 2 out]
      n94 = call-poly <vilib>:"NT Write Value.vi"("String Array"=string[] ["New Name"], "Name"="DB/Button Names") -> ()  [unwired: 9 in, 1 out]
      n95 = disable-structure shown="Disabled" {
        frame Disabled {
          (unwired) 0.000147 ("Scaling factor (s/in)")
          n96 = call-poly <vilib>:"WPI_UltrasonicOpen.vi"("DIO Channel"=FPGA_DIOChannel."DIO 9") -> ("error out"=w265:errorcluster, "SonarMB1010DigitalDevRef"=w266:T32)  [unwired: 9 in]
          n97 = call-poly <vilib>:"WPI_UltrasonicRefNum Registry Set.vi"("error in (no error)"=w265, "refnum name"="RangeFinder", "SonarMB1010DigitalDevRef"=w266) -> ()  [unwired: 7 in, 2 out]
        }
        frame Enabled {
        }
      }
      n98 = call <vilib>:"CTRE_Phoenix_TalonSRX_Open.vi"("Invert"=TRUE, "Device Number"=u8 1) -> ("CAN Talon SRX Ref"=w178:T23)  [unwired: 8 in, 1 out]
      n99 = call-poly <vilib>:"NT Write Value.vi"("String Array"=string[] ["1-AutoScale", "2-Auto", "3-AutoScale", "Exist", "1-Scale\n1-Switcch\n3-Scale\n3-Switch", "1-Switch", "3-Scale", "3-Switch", "MiniExist", "1-AutoSwitch", "3-AutoSwitch"], "Name"="Auto List") -> ()  [unwired: 9 in, 1 out]
      n100 = call <vilib>:"CTRE_Phoenix_MotorControl_RefNumRegistrySet.vi"("refnum name"="DriveRight", "PhoenixMotorControlDevRef"=w178) -> ("PhoenixMotorControlDevRef"=w157:T23)  [unwired: 8 in, 1 out]
      n101 = call <vilib>:"CTRE_Phoenix_TalonSRX_Open.vi"("Invert"=TRUE, "Device Number"=u8 3) -> ("CAN Talon SRX Ref"=w219:T23)  [unwired: 8 in, 1 out]
      n102 = call <vilib>:"CTRE_Phoenix_TalonSRX_Open.vi"("Invert"=TRUE, "Device Number"=u8 5) -> ("CAN Talon SRX Ref"=w200:T23)  [unwired: 8 in, 1 out]
      n103 = call <vilib>:"WPI_RelayOpen.vi"("Relay Channel"=FPGA_DIORelayChannel."Relay 0") -> ("error out"=w191:errorcluster, "RelayDevRef"=w190:T34)  [unwired: 9 in]
      n104 = call <vilib>:"CTRE_Phoenix_MotorControl_Follow.vi"("Master Controller to Follow"=w157, "PhoenixMotorControlDevRef"=w200) -> ()  [unwired: 8 in, 2 out]
      n105 = call <vilib>:"CTRE_Phoenix_MotorControl_Follow.vi"("Master Controller to Follow"=w157, "PhoenixMotorControlDevRef"=w219) -> ()  [unwired: 8 in, 2 out]
      n106 = call <vilib>:"WPI_CompressorOpen.vi"("Pneumatics Control Module (0)"=u8 13) -> ("CompressorDevRef"=w224:T21, "error out"=w225:errorcluster)  [unwired: 13 in]
      n107 = call <vilib>:"WPI_RelayRefNum Registry Set.vi"("error in (no error)"=w191, "refnum name"="FanControl", "RelayDevRef"=w190) -> ()  [unwired: 7 in, 2 out]
      n108 = call <vilib>:"CTRE_Phoenix_TalonSRX_Open.vi"("Invert"=FALSE, "Device Number"=u8 7) -> ("error out"=w215:errorcluster, "CAN Talon SRX Ref"=w214:T23)  [unwired: 8 in]
      n109 = call <vilib>:"CTRE_Phoenix_MotorControl_ConfigOpenLoopRamp.vi"("secondsFromNeutralToFull"=w154, "PhoenixMotorControlDevRef"=w157) -> ()  [unwired: 8 in, 2 out]
      n110 = call <vilib>:"CTRE_Phoenix_MotorControl_SetNeutralMode.vi"("Motor Control Neutral Mode"=CTRE_Phoenix_MotorControl_NeutralMode."Override to Brake", "PhoenixMotorControlDevRef"=w157) -> ()  [unwired: 8 in, 2 out]
      n111 = call <vilib>:"CTRE_Phoenix_MotorControl_ConfigSelectedFeedbackSensor_Enhanced.vi"("Feedback Device"=w176, "PhoenixMotorControlDevRef"=w157) -> ()  [unwired: 8 in, 2 out]
      n112 = disable-structure shown="Disabled" {
        frame Disabled {
          w269 = 1.0  # Sample Rate (ms)
          n113 = call-poly <vilib>:"WPI_GyroOpen.vi"("Sample Rate (Hz)"=w269, "SPI Bus"=spi_bus."SPI On-Board, CS0") -> ("GyroDevRef"=w271:T36)  [unwired: 7 in, 2 out]
          n114 = call <vilib>:"WPI_GyroReset.vi"("GyroDevRef"=w271) -> ("GyroDevRef"=w270:T36)  [unwired: 9 in, 1 out]
          n115 = call <vilib>:"WPI_GyroRefNum Registry Set.vi"("refnum name"="Gyro2", "GyroDevRef"=w270) -> ()  [unwired: 8 in, 2 out]
        }
        frame Enabled {
        }
      }
      n116 = call <vilib>:"WPI_CompressorRefNum Registry Set.vi"("error in (no error)"=w225, "refnum name"="Compressor", "CompressorDevRef"=w224) -> ()  [unwired: 7 in, 2 out]
      n117 = call <vilib>:"CTRE_Phoenix_TalonSRX_Open.vi"("Invert"=FALSE, "Device Number"=u8 8) -> ("error out"=w210:errorcluster, "CAN Talon SRX Ref"=w209:T23)  [unwired: 8 in]
      n118 = call <vilib>:"CTRE_Phoenix_MotorControl_RefNumRegistrySet.vi"("error in (no error)"=w215, "refnum name"="Lifter", "PhoenixMotorControlDevRef"=w214) -> ("error out"=w192:errorcluster, "PhoenixMotorControlDevRef"=w169:T23)  [unwired: 7 in]
      n119 = call <vilib>:"CTRE_Phoenix_TalonSRX_Open.vi"("Invert"=FALSE, "Device Number"=u8 2) -> ("CAN Talon SRX Ref"=w177:T23)  [unwired: 8 in, 1 out]
      n120 = call <vilib>:"CTRE_Phoenix_MotorControl_Follow.vi"("error in (no error)"=w210, "Master Controller to Follow"=w169, "PhoenixMotorControlDevRef"=w209) -> ("error out"=w196:errorcluster, "PhoenixMotorControlDevRef"=w194:T23)  [unwired: 7 in]
      n121 = call <vilib>:"CTRE_Phoenix_MotorControl_RefNumRegistrySet.vi"("refnum name"="DriveLeft", "PhoenixMotorControlDevRef"=w177) -> ("PhoenixMotorControlDevRef"=w156:T23)  [unwired: 8 in, 1 out]
      n122 = call <vilib>:"CTRE_Phoenix_TalonSRX_Open.vi"("Invert"=FALSE, "Device Number"=u8 4) -> ("CAN Talon SRX Ref"=w197:T23)  [unwired: 8 in, 1 out]
      n123 = call <vilib>:"CTRE_Phoenix_TalonSRX_Open.vi"("Invert"=FALSE, "Device Number"=u8 6) -> ("CAN Talon SRX Ref"=w242:T23)  [unwired: 8 in, 1 out]
      n124 = call <vilib>:"CTRE_Phoenix_MotorControl_OverrideLimitSwitchesEnable.vi"("PhoenixMotorControlDevRef"=w169, "Override Limit Switch Enable?"=TRUE, "error in (no error)"=w192) -> ()  [unwired: 11 in, 2 out]
      n125 = call <vilib>:"CTRE_Phoenix_MotorControl_ConfigSelectedFeedbackSensor_Enhanced.vi"("pidLoopIdx"=0, "Feedback Device"=w174, "PhoenixMotorControlDevRef"=w169) -> ()  [unwired: 7 in, 2 out]
      n126 = call <vilib>:"CTRE_Phoenix_MotorControl_Follow.vi"("Master Controller to Follow"=w156, "PhoenixMotorControlDevRef"=w197) -> ()  [unwired: 8 in, 2 out]
      n127 = call <vilib>:"CTRE_Phoenix_MotorControl_Follow.vi"("Master Controller to Follow"=w156, "PhoenixMotorControlDevRef"=w242) -> ()  [unwired: 8 in, 2 out]
      n128 = call <vilib>:"CTRE_Phoenix_MotorControl_SetNeutralMode.vi"("Motor Control Neutral Mode"=CTRE_Phoenix_MotorControl_NeutralMode."Override to Brake", "PhoenixMotorControlDevRef"=w156) -> ()  [unwired: 8 in, 2 out]
      n129 = call <vilib>:"CTRE_Phoenix_MotorControl_ConfigOpenLoopRamp.vi"("secondsFromNeutralToFull"=w154, "PhoenixMotorControlDevRef"=w156) -> ()  [unwired: 8 in, 2 out]
      n130 = call <vilib>:"CTRE_Phoenix_MotorControl_ConfigSelectedFeedbackSensor_Enhanced.vi"("Feedback Device"=w175, "PhoenixMotorControlDevRef"=w156) -> ()  [unwired: 8 in, 2 out]
      n131 = call <vilib>:"CTRE_Phoenix_MotorControl_RefNumRegistrySet.vi"("error in (no error)"=w196, "refnum name"="LifterSlave", "PhoenixMotorControlDevRef"=w194) -> ()  [unwired: 7 in, 2 out]
      n132 = call-poly <vilib>:"CTRE_PigeonIMU_Open.vi"("Device Number"=u8 12) -> ("error out"=w222:errorcluster, "PigeonIMUDevRef"=w221:T28)  [unwired: 9 in]
      n133 = call <vilib>:"CTRE_Phoenix_MotorControl_EnableCurrentLimit.vi"("Enable Current Limit?"=w155, "PhoenixMotorControlDevRef"=w157) -> ("PhoenixMotorControlDevRef"=w164:T23)  [unwired: 8 in, 1 out]
      n134 = call <vilib>:"CTRE_Phoenix_MotorControl_EnableCurrentLimit.vi"("Enable Current Limit?"=w155, "PhoenixMotorControlDevRef"=w156) -> ("PhoenixMotorControlDevRef"=w162:T23)  [unwired: 8 in, 1 out]
      n135 = call <vilib>:"CTRE_Phoenix_MotorControl_SetNeutralMode.vi"("Motor Control Neutral Mode"=CTRE_Phoenix_MotorControl_NeutralMode."Override to Brake", "PhoenixMotorControlDevRef"=w169) -> ()  [unwired: 8 in, 2 out]
      n136 = call-poly <vilib>:"WPI_RobotDriveOpen2Motor.vi"("Right Motor Dev Ref"=w157, "Left Motor Dev Ref"=w156) -> ("error out"=w249:errorcluster, "RobotDriveDevRef"=w248:T27)  [unwired: 8 in]
      n137 = call <vilib>:"CTRE_Phoenix_MotorControl_ConfigContinuousCurrentLimit.vi"("Continuous Current Limit (Amps)"=w160, "PhoenixMotorControlDevRef"=w164) -> ("PhoenixMotorControlDevRef"=w163:T23)  [unwired: 8 in, 1 out]
      n138 = call <vilib>:"CTRE_Phoenix_MotorControl_ConfigContinuousCurrentLimit.vi"("Continuous Current Limit (Amps)"=w160, "PhoenixMotorControlDevRef"=w162) -> ("PhoenixMotorControlDevRef"=w161:T23)  [unwired: 8 in, 1 out]
      n139 = call <vilib>:"CTRE_PigeonIMU_RefNumRegistrySet.vi"("error in (no error)"=w222, "refnum name"="Gyro", "PigeonIMUDevRef"=w221) -> ("error out"=w167:errorcluster, "PigeonIMUDevRef"=w168:T28)  [unwired: 7 in]
      n140 = call <vilib>:"CTRE_Phoenix_MotorControl_ConfigPeakCurrentLimit.vi"("Peak Current Maximum Duration (ms)"=w158, "Peak Current (Amps)"=w159, "PhoenixMotorControlDevRef"=w163) -> ()  [unwired: 7 in, 2 out]
      n141 = call <vilib>:"CTRE_Phoenix_MotorControl_ConfigPeakCurrentLimit.vi"("Peak Current Maximum Duration (ms)"=w158, "Peak Current (Amps)"=w159, "PhoenixMotorControlDevRef"=w161) -> ()  [unwired: 7 in, 2 out]
      n142 = call <vilib>:"WPI_RobotDriveRefNum Registry Set.vi"("error in (no error)"=w249, "refnum name"="RobotDrive", "RobotDriveDevRef"=w248) -> ()  [unwired: 7 in, 2 out]
      n143 = call <vilib>:"CTRE_PigeonIMU_SetYaw.vi"("error in (no error)"=w167, "Value"=0.0, "PigeonIMUDevRef"=w168) -> ()  [unwired: 7 in, 2 out]
      n144 = call <vilib>:"CTRE_PigeonIMU_SetFusedHeading.vi"("error in (no error)"=w167, "Value"=0.0, "PigeonIMUDevRef 2"=w168) -> ()  [unwired: 7 in, 2 out]
      "error out 2" <- "error in 2"
    }
    frame "2018P Drew" {
      w323 = 250  # Peak Current Maximum Duration (ms)
      w324 = 50  # Peak Current (Amps)
      w325 = 40  # Continuous Current Limit (Amps)
      w320 = TRUE ("Enable Current Limit?")
      w339 = T30 0 items=["None"=-1, "QuadEncoder"=0, "Analog"=2, "Tachometer"=4, "Pulse Width Encoded Position"=8, "Sensor Sum (S0 + S1)"=9, "Sensor Difference (D0 - D1)"=10, "Remote Source 0"=11, "Remote Source 1"=12, "Software Emulated"=15] ("Feedback Device")
      w340 = T30 0 items=["None"=-1, "QuadEncoder"=0, "Analog"=2, "Tachometer"=4, "Pulse Width Encoded Position"=8, "Sensor Sum (S0 + S1)"=9, "Sensor Difference (D0 - D1)"=10, "Remote Source 0"=11, "Remote Source 1"=12, "Software Emulated"=15] ("Feedback Device")
      w341 = T30 0 items=["None"=-1, "QuadEncoder"=0, "Analog"=2, "Tachometer"=4, "Pulse Width Encoded Position"=8, "Sensor Sum (S0 + S1)"=9, "Sensor Difference (D0 - D1)"=10, "Remote Source 0"=11, "Remote Source 1"=12, "Software Emulated"=15] ("Feedback Device")
      w319 = 0.25  # secondsFromNeutralToFull
      (unwired) "This VI is called before others so you can setup for execution.\n\nThe data and I/O allocated here will be made available to the loops for camera, periodic, and to the Auto and TeleOp VIs. To add more I/O, use an Open VI followed by a Refnum Registry Set VI.  Use a Refnum Registry Get VI in the other locations.\n\nYou may also want to use global variables to communicate between parallel loops."
      # "Testing"
      # "1-Auto\n2-Auto\n3-Auto\nExist"
      # "3-Scale\n3-Switch\n1-Scale\n1-Switch"
      # "Forward"
      # "Reverse"
      # "The Drive tab of the default dashboard displays the contents of the\nAuto List variable. When the user selects a value, it will be written to\nthe Auto Selector variable. You may want to use this, along with other\ndashboard inputs, to let drivers define the robot's autonomous\nbehavior."
      # "The code below shows how to give controls on the\nBasic tab more specific names. You can set\nButton Names, LED Names, Slider Names,\nand String Names."
      # "initialize a joystick"
      # "Until the communications specify the mode,\ninitialize it to a safe value."
      n145 = call <vilib>:"WPI_AnalogChannelOpen.vi"("Analog Channel"=FPGA_AIChannel."AI 0") -> ("error out"=w315:errorcluster, "AIDeviceRef"=w316:T31)  [unwired: 9 in]
      n146 = call <vilib>:"WPI_JoystickOpen.vi"("JoystickDevice"=WPI_JoystickDeviceEnum."USB 0") -> ("JoystickDevRef"=w426:T10)  [unwired: 10 in]
      n147 = call <vilib>:"WPI_JoystickOpen.vi"("JoystickDevice"=WPI_JoystickDeviceEnum."USB 1") -> ("JoystickDevRef"=w382:T10)  [unwired: 10 in]
      n148 = call <vilib>:"WPI_DigitalInputOpen.vi"("DIO Channel"=FPGA_DIOChannel."DIO 6") -> ("error out"=w305:errorcluster, "DigitalInputDevRef"=w304:T11)  [unwired: 9 in]
      n149 = call <vilib>:"WPI_DigitalInputOpen.vi"("DIO Channel"=FPGA_DIOChannel."DIO 3") -> ("error out"=w308:errorcluster, "DigitalInputDevRef"=w307:T11)  [unwired: 9 in]
      n150 = call <vilib>:"WPI_DigitalInputOpen.vi"("DIO Channel"=FPGA_DIOChannel."DIO 0") -> ("error out"=w311:errorcluster, "DigitalInputDevRef"=w310:T11)  [unwired: 9 in]
      n151 = call <vilib>:"WPI_AnalogChannelRefNum Registry Set.vi"("error in (no error)"=w315, "refnum name"="PressureSensor", "AIDeviceRef"=w316) -> ()  [unwired: 7 in, 2 out]
      n152 = call <vilib>:"WPI_DigitalInputRefNum Registry Set.vi"("error in (no error)"=w305, "refnum name"="Selector6", "DigitalInputDevRef"=w304) -> ()  [unwired: 7 in, 2 out]
      n153 = call <vilib>:"WPI_JoystickRefNum Registry Set.vi"("refnum name"="Joystick 1", "JoystickDevRef"=w382) -> ()  [unwired: 8 in, 2 out]
      n154 = call <vilib>:"WPI_DigitalInputRefNum Registry Set.vi"("error in (no error)"=w308, "refnum name"="Selector3", "DigitalInputDevRef"=w307) -> ()  [unwired: 7 in, 2 out]
      n155 = call <vilib>:"WPI_DigitalInputRefNum Registry Set.vi"("error in (no error)"=w311, "refnum name"="Selector0", "DigitalInputDevRef"=w310) -> ()  [unwired: 7 in, 2 out]
      n156 = call <vilib>:"WPI_JoystickRefNum Registry Set.vi"("refnum name"="Joystick 0", "JoystickDevRef"=w426) -> ()  [unwired: 8 in, 2 out]
      n157 = call <vilib>:"WPI_DigitalInputOpen.vi"("DIO Channel"=FPGA_DIOChannel."DIO 7") -> ("error out"=w302:errorcluster, "DigitalInputDevRef"=w301:T11)  [unwired: 9 in]
      n158 = call <vilib>:"WPI_DigitalInputOpen.vi"("DIO Channel"=FPGA_DIOChannel."DIO 4") -> ("error out"=w299:errorcluster, "DigitalInputDevRef"=w298:T11)  [unwired: 9 in]
      n159 = call <vilib>:"WPI_DigitalInputOpen.vi"("DIO Channel"=FPGA_DIOChannel."DIO 1") -> ("error out"=w296:errorcluster, "DigitalInputDevRef"=w295:T11)  [unwired: 9 in]
      n160 = global write "Robot Global Data.vi" "Robot Mode"(WPI_DriverStationRobotMode2."Autonomous Disabled" ("Robot Mode")) -> ()
      n161 = call <vilib>:"WPI_DigitalInputRefNum Registry Set.vi"("error in (no error)"=w302, "refnum name"="Selector7", "DigitalInputDevRef"=w301) -> ()  [unwired: 7 in, 2 out]
      n162 = call <vilib>:"WPI_DigitalInputRefNum Registry Set.vi"("error in (no error)"=w299, "refnum name"="Selector4", "DigitalInputDevRef"=w298) -> ()  [unwired: 7 in, 2 out]
      n163 = call-poly <vilib>:"WPI_SolenoidOpen.vi"("Solenoid Channel"=WPI_SolenoidChannel."Solenoid 7" ("Forward Solenoid Channel"), "Pneumatics Control Module (0)"=u8 13) -> ("error out"=w371:errorcluster, "SolenoidDevRef"=w370:T20)  [unwired: 8 in]
      n164 = call <vilib>:"WPI_DigitalInputRefNum Registry Set.vi"("error in (no error)"=w296, "refnum name"="Selector1", "DigitalInputDevRef"=w295) -> ()  [unwired: 7 in, 2 out]
      n165 = call-poly <vilib>:"WPI_SolenoidOpen.vi"("Solenoid Channel"=WPI_SolenoidChannel."Solenoid 5" ("Forward Solenoid Channel"), "Pneumatics Control Module (0)"=u8 13) -> ("error out"=w398:errorcluster, "SolenoidDevRef"=w397:T20)  [unwired: 8 in]
      n166 = call-poly <vilib>:"WPI_SolenoidOpen.vi"("Solenoid Channel"=WPI_SolenoidChannel."Solenoid 0" ("Forward Solenoid Channel"), "Pneumatics Control Module (0)"=u8 13) -> ("error out"=w402:errorcluster, "SolenoidDevRef"=w401:T20)  [unwired: 8 in]
      n167 = call-poly <vilib>:"WPI_SolenoidOpen.vi"("Solenoid Channel"=WPI_SolenoidChannel."Solenoid 1" ("Forward Solenoid Channel"), "Pneumatics Control Module (0)"=u8 13) -> ("error out"=w406:errorcluster, "SolenoidDevRef"=w405:T20)  [unwired: 8 in]
      n168 = call-poly <vilib>:"WPI_SolenoidSet.vi"("Value"=WPI_SolenoidValue."Off", "SolenoidDevRef"=w397) -> ("SolenoidDevRef"=w347:T20)  [unwired: 8 in, 1 out]
      n169 = call-poly <vilib>:"WPI_SolenoidSet.vi"("Value"=WPI_SolenoidValue."Off", "SolenoidDevRef"=w401) -> ("SolenoidDevRef"=w351:T20)  [unwired: 8 in, 1 out]
      n170 = call <vilib>:"WPI_DigitalInputOpen.vi"("DIO Channel"=FPGA_DIOChannel."DIO 2") -> ("error out"=w293:errorcluster, "DigitalInputDevRef"=w292:T11)  [unwired: 9 in]
      n171 = call <vilib>:"WPI_DigitalInputOpen.vi"("DIO Channel"=FPGA_DIOChannel."DIO 8") -> ("error out"=w287:errorcluster, "DigitalInputDevRef"=w286:T11)  [unwired: 9 in]
      n172 = call-poly <vilib>:"WPI_SolenoidSet.vi"("Value"=WPI_SolenoidValue."Off", "SolenoidDevRef"=w370) -> ("SolenoidDevRef"=w346:T20)  [unwired: 8 in, 1 out]
      n173 = call <vilib>:"WPI_DigitalInputOpen.vi"("DIO Channel"=FPGA_DIOChannel."DIO 5") -> ("error out"=w290:errorcluster, "DigitalInputDevRef"=w289:T11)  [unwired: 9 in]
      n174 = call-poly <vilib>:"WPI_SolenoidSet.vi"("Value"=WPI_SolenoidValue."Off", "SolenoidDevRef"=w405) -> ("SolenoidDevRef"=w350:T20)  [unwired: 8 in, 1 out]
      n175 = call <vilib>:"WPI_DigitalInputRefNum Registry Set.vi"("error in (no error)"=w293, "refnum name"="Selector2", "DigitalInputDevRef"=w292) -> ()  [unwired: 7 in, 2 out]
      n176 = call <vilib>:"WPI_DigitalInputRefNum Registry Set.vi"("error in (no error)"=w287, "refnum name"="Selector8", "DigitalInputDevRef"=w286) -> ()  [unwired: 7 in, 2 out]
      n177 = call <vilib>:"WPI_DigitalInputRefNum Registry Set.vi"("error in (no error)"=w290, "refnum name"="Selector5", "DigitalInputDevRef"=w289) -> ()  [unwired: 7 in, 2 out]
      n178 = call <vilib>:"WPI_SolenoidRefNum Registry Set.vi"("error in (no error)"=w406, "refnum name"="ArmSolenoid", "SolenoidDevRef"=w350) -> ()  [unwired: 7 in, 2 out]
      n179 = call <vilib>:"WPI_SolenoidRefNum Registry Set.vi"("error in (no error)"=w398, "refnum name"="Shifter", "SolenoidDevRef"=w347) -> ()  [unwired: 7 in, 2 out]
      n180 = call <vilib>:"WPI_SolenoidRefNum Registry Set.vi"("error in (no error)"=w402, "refnum name"="Gripper", "SolenoidDevRef"=w351) -> ()  [unwired: 7 in, 2 out]
      n181 = call <vilib>:"WPI_SolenoidRefNum Registry Set.vi"("error in (no error)"=w371, "refnum name"="LifterShifter", "SolenoidDevRef"=w346) -> ()  [unwired: 7 in, 2 out]
      n182 = call <vilib>:"WPI_DigitalInputOpen.vi"("DIO Channel"=FPGA_DIOChannel."DIO 9") -> ("error out"=w275:errorcluster, "DigitalInputDevRef"=w274:T11)  [unwired: 9 in]
      n183 = call <vilib>:"WPI_DigitalInputRefNum Registry Set.vi"("error in (no error)"=w275, "refnum name"="Selector9", "DigitalInputDevRef"=w274) -> ()  [unwired: 7 in, 2 out]
      n184 = call-poly <vilib>:"NT Write Value.vi"("String Array"=string[] ["New Name"], "Name"="DB/Button Names") -> ()  [unwired: 9 in, 1 out]
      n185 = disable-structure shown="Disabled" {
        frame Disabled {
          (unwired) 0.000147 ("Scaling factor (s/in)")
          n186 = call-poly <vilib>:"WPI_UltrasonicOpen.vi"("DIO Channel"=FPGA_DIOChannel."DIO 9") -> ("error out"=w430:errorcluster, "SonarMB1010DigitalDevRef"=w431:T32)  [unwired: 9 in]
          n187 = call-poly <vilib>:"WPI_UltrasonicRefNum Registry Set.vi"("error in (no error)"=w430, "refnum name"="RangeFinder", "SonarMB1010DigitalDevRef"=w431) -> ()  [unwired: 7 in, 2 out]
        }
        frame Enabled {
        }
      }
      n188 = call <vilib>:"CTRE_Phoenix_TalonSRX_Open.vi"("Invert"=TRUE, "Device Number"=u8 1) -> ("CAN Talon SRX Ref"=w343:T23)  [unwired: 8 in, 1 out]
      n189 = call-poly <vilib>:"NT Write Value.vi"("String Array"=string[] ["1-AutoScale", "2-Auto", "3-AutoScale", "Exist", "1-Scale\n1-Switcch\n3-Scale\n3-Switch", "1-Switch", "3-Scale", "3-Switch", "MiniExist", "1-AutoSwitch", "3-AutoSwitch"], "Name"="Auto List") -> ()  [unwired: 9 in, 1 out]
      n190 = call <vilib>:"CTRE_Phoenix_MotorControl_RefNumRegistrySet.vi"("refnum name"="DriveRight", "PhoenixMotorControlDevRef"=w343) -> ("PhoenixMotorControlDevRef"=w322:T23)  [unwired: 8 in, 1 out]
      n191 = call <vilib>:"CTRE_Phoenix_TalonSRX_Open.vi"("Invert"=TRUE, "Device Number"=u8 3) -> ("CAN Talon SRX Ref"=w384:T23)  [unwired: 8 in, 1 out]
      n192 = call <vilib>:"CTRE_Phoenix_TalonSRX_Open.vi"("Invert"=TRUE, "Device Number"=u8 5) -> ("CAN Talon SRX Ref"=w365:T23)  [unwired: 8 in, 1 out]
      n193 = call <vilib>:"WPI_RelayOpen.vi"("Relay Channel"=FPGA_DIORelayChannel."Relay 0") -> ("error out"=w356:errorcluster, "RelayDevRef"=w355:T34)  [unwired: 9 in]
      n194 = call <vilib>:"CTRE_Phoenix_MotorControl_Follow.vi"("Master Controller to Follow"=w322, "PhoenixMotorControlDevRef"=w365) -> ()  [unwired: 8 in, 2 out]
      n195 = call <vilib>:"CTRE_Phoenix_MotorControl_Follow.vi"("Master Controller to Follow"=w322, "PhoenixMotorControlDevRef"=w384) -> ()  [unwired: 8 in, 2 out]
      n196 = call <vilib>:"WPI_CompressorOpen.vi"("Pneumatics Control Module (0)"=u8 13) -> ("CompressorDevRef"=w389:T21, "error out"=w390:errorcluster)  [unwired: 13 in]
      n197 = call <vilib>:"WPI_RelayRefNum Registry Set.vi"("error in (no error)"=w356, "refnum name"="FanControl", "RelayDevRef"=w355) -> ()  [unwired: 7 in, 2 out]
      n198 = call <vilib>:"CTRE_Phoenix_TalonSRX_Open.vi"("Invert"=FALSE, "Device Number"=u8 7) -> ("error out"=w380:errorcluster, "CAN Talon SRX Ref"=w379:T23)  [unwired: 8 in]
      n199 = call <vilib>:"CTRE_Phoenix_MotorControl_ConfigOpenLoopRamp.vi"("secondsFromNeutralToFull"=w319, "PhoenixMotorControlDevRef"=w322) -> ()  [unwired: 8 in, 2 out]
      n200 = call <vilib>:"CTRE_Phoenix_MotorControl_SetNeutralMode.vi"("Motor Control Neutral Mode"=CTRE_Phoenix_MotorControl_NeutralMode."Override to Brake", "PhoenixMotorControlDevRef"=w322) -> ()  [unwired: 8 in, 2 out]
      n201 = call <vilib>:"CTRE_Phoenix_MotorControl_ConfigSelectedFeedbackSensor_Enhanced.vi"("Feedback Device"=w341, "PhoenixMotorControlDevRef"=w322) -> ()  [unwired: 8 in, 2 out]
      n202 = disable-structure shown="Disabled" {
        frame Disabled {
          w434 = 1.0  # Sample Rate (ms)
          n203 = call-poly <vilib>:"WPI_GyroOpen.vi"("Sample Rate (Hz)"=w434, "SPI Bus"=spi_bus."SPI On-Board, CS0") -> ("GyroDevRef"=w436:T36)  [unwired: 7 in, 2 out]
          n204 = call <vilib>:"WPI_GyroReset.vi"("GyroDevRef"=w436) -> ("GyroDevRef"=w435:T36)  [unwired: 9 in, 1 out]
          n205 = call <vilib>:"WPI_GyroRefNum Registry Set.vi"("refnum name"="Gyro2", "GyroDevRef"=w435) -> ()  [unwired: 8 in, 2 out]
        }
        frame Enabled {
        }
      }
      n206 = call <vilib>:"WPI_CompressorRefNum Registry Set.vi"("error in (no error)"=w390, "refnum name"="Compressor", "CompressorDevRef"=w389) -> ()  [unwired: 7 in, 2 out]
      n207 = call <vilib>:"CTRE_Phoenix_TalonSRX_Open.vi"("Invert"=FALSE, "Device Number"=u8 8) -> ("error out"=w375:errorcluster, "CAN Talon SRX Ref"=w374:T23)  [unwired: 8 in]
      n208 = call <vilib>:"CTRE_Phoenix_MotorControl_RefNumRegistrySet.vi"("error in (no error)"=w380, "refnum name"="Lifter", "PhoenixMotorControlDevRef"=w379) -> ("error out"=w357:errorcluster, "PhoenixMotorControlDevRef"=w334:T23)  [unwired: 7 in]
      n209 = call <vilib>:"CTRE_Phoenix_TalonSRX_Open.vi"("Invert"=FALSE, "Device Number"=u8 2) -> ("CAN Talon SRX Ref"=w342:T23)  [unwired: 8 in, 1 out]
      n210 = call <vilib>:"CTRE_Phoenix_MotorControl_Follow.vi"("error in (no error)"=w375, "Master Controller to Follow"=w334, "PhoenixMotorControlDevRef"=w374) -> ("error out"=w361:errorcluster, "PhoenixMotorControlDevRef"=w359:T23)  [unwired: 7 in]
      n211 = call <vilib>:"CTRE_Phoenix_MotorControl_RefNumRegistrySet.vi"("refnum name"="DriveLeft", "PhoenixMotorControlDevRef"=w342) -> ("PhoenixMotorControlDevRef"=w321:T23)  [unwired: 8 in, 1 out]
      n212 = call <vilib>:"CTRE_Phoenix_TalonSRX_Open.vi"("Invert"=FALSE, "Device Number"=u8 4) -> ("CAN Talon SRX Ref"=w362:T23)  [unwired: 8 in, 1 out]
      n213 = call <vilib>:"CTRE_Phoenix_TalonSRX_Open.vi"("Invert"=FALSE, "Device Number"=u8 6) -> ("CAN Talon SRX Ref"=w407:T23)  [unwired: 8 in, 1 out]
      n214 = call <vilib>:"CTRE_Phoenix_MotorControl_OverrideLimitSwitchesEnable.vi"("PhoenixMotorControlDevRef"=w334, "Override Limit Switch Enable?"=TRUE, "error in (no error)"=w357) -> ()  [unwired: 11 in, 2 out]
      n215 = call <vilib>:"CTRE_Phoenix_MotorControl_ConfigSelectedFeedbackSensor_Enhanced.vi"("pidLoopIdx"=0, "Feedback Device"=w339, "PhoenixMotorControlDevRef"=w334) -> ()  [unwired: 7 in, 2 out]
      n216 = call <vilib>:"CTRE_Phoenix_MotorControl_Follow.vi"("Master Controller to Follow"=w321, "PhoenixMotorControlDevRef"=w362) -> ()  [unwired: 8 in, 2 out]
      n217 = call <vilib>:"CTRE_Phoenix_MotorControl_Follow.vi"("Master Controller to Follow"=w321, "PhoenixMotorControlDevRef"=w407) -> ()  [unwired: 8 in, 2 out]
      n218 = call <vilib>:"CTRE_Phoenix_MotorControl_SetNeutralMode.vi"("Motor Control Neutral Mode"=CTRE_Phoenix_MotorControl_NeutralMode."Override to Brake", "PhoenixMotorControlDevRef"=w321) -> ()  [unwired: 8 in, 2 out]
      n219 = call <vilib>:"CTRE_Phoenix_MotorControl_ConfigOpenLoopRamp.vi"("secondsFromNeutralToFull"=w319, "PhoenixMotorControlDevRef"=w321) -> ()  [unwired: 8 in, 2 out]
      n220 = call <vilib>:"CTRE_Phoenix_MotorControl_ConfigSelectedFeedbackSensor_Enhanced.vi"("Feedback Device"=w340, "PhoenixMotorControlDevRef"=w321) -> ()  [unwired: 8 in, 2 out]
      n221 = call <vilib>:"CTRE_Phoenix_MotorControl_RefNumRegistrySet.vi"("error in (no error)"=w361, "refnum name"="LifterSlave", "PhoenixMotorControlDevRef"=w359) -> ()  [unwired: 7 in, 2 out]
      n222 = call-poly <vilib>:"CTRE_PigeonIMU_Open.vi"("Device Number"=u8 12) -> ("error out"=w387:errorcluster, "PigeonIMUDevRef"=w386:T28)  [unwired: 9 in]
      n223 = call <vilib>:"CTRE_Phoenix_MotorControl_EnableCurrentLimit.vi"("Enable Current Limit?"=w320, "PhoenixMotorControlDevRef"=w322) -> ("PhoenixMotorControlDevRef"=w329:T23)  [unwired: 8 in, 1 out]
      n224 = call <vilib>:"CTRE_Phoenix_MotorControl_EnableCurrentLimit.vi"("Enable Current Limit?"=w320, "PhoenixMotorControlDevRef"=w321) -> ("PhoenixMotorControlDevRef"=w327:T23)  [unwired: 8 in, 1 out]
      n225 = call <vilib>:"CTRE_Phoenix_MotorControl_SetNeutralMode.vi"("Motor Control Neutral Mode"=CTRE_Phoenix_MotorControl_NeutralMode."Override to Brake", "PhoenixMotorControlDevRef"=w334) -> ()  [unwired: 8 in, 2 out]
      n226 = call-poly <vilib>:"WPI_RobotDriveOpen2Motor.vi"("Right Motor Dev Ref"=w322, "Left Motor Dev Ref"=w321) -> ("error out"=w414:errorcluster, "RobotDriveDevRef"=w413:T27)  [unwired: 8 in]
      n227 = call <vilib>:"CTRE_Phoenix_MotorControl_ConfigContinuousCurrentLimit.vi"("Continuous Current Limit (Amps)"=w325, "PhoenixMotorControlDevRef"=w329) -> ("PhoenixMotorControlDevRef"=w328:T23)  [unwired: 8 in, 1 out]
      n228 = call <vilib>:"CTRE_Phoenix_MotorControl_ConfigContinuousCurrentLimit.vi"("Continuous Current Limit (Amps)"=w325, "PhoenixMotorControlDevRef"=w327) -> ("PhoenixMotorControlDevRef"=w326:T23)  [unwired: 8 in, 1 out]
      n229 = call <vilib>:"CTRE_PigeonIMU_RefNumRegistrySet.vi"("error in (no error)"=w387, "refnum name"="Gyro", "PigeonIMUDevRef"=w386) -> ("error out"=w332:errorcluster, "PigeonIMUDevRef"=w333:T28)  [unwired: 7 in]
      n230 = call <vilib>:"CTRE_Phoenix_MotorControl_ConfigPeakCurrentLimit.vi"("Peak Current Maximum Duration (ms)"=w323, "Peak Current (Amps)"=w324, "PhoenixMotorControlDevRef"=w328) -> ()  [unwired: 7 in, 2 out]
      n231 = call <vilib>:"CTRE_Phoenix_MotorControl_ConfigPeakCurrentLimit.vi"("Peak Current Maximum Duration (ms)"=w323, "Peak Current (Amps)"=w324, "PhoenixMotorControlDevRef"=w326) -> ()  [unwired: 7 in, 2 out]
      n232 = call <vilib>:"WPI_RobotDriveRefNum Registry Set.vi"("error in (no error)"=w414, "refnum name"="RobotDrive", "RobotDriveDevRef"=w413) -> ()  [unwired: 7 in, 2 out]
      n233 = call <vilib>:"CTRE_PigeonIMU_SetYaw.vi"("error in (no error)"=w332, "Value"=0.0, "PigeonIMUDevRef"=w333) -> ()  [unwired: 7 in, 2 out]
      n234 = call <vilib>:"CTRE_PigeonIMU_SetFusedHeading.vi"("error in (no error)"=w332, "Value"=0.0, "PigeonIMUDevRef 2"=w333) -> ()  [unwired: 7 in, 2 out]
      "error out 3" <- "error in 3"
    }
  }
